vi "Notifier Release.vi"(8 "error in (no error)":errorcluster, 11 "Messaging in":refnum<class "Messaging.lvclass">) -> (0 "error out":errorcluster, 3 "Messaging out":refnum<class "Messaging.lvclass">)   [LabVIEW 2023, in "MessagingModule.lvlib" / "Messaging.lvclass"]
uses:
  Messaging.lvclass
  Messaging.lvclass/Messaging.ctl
  MessagingModule.lvlib
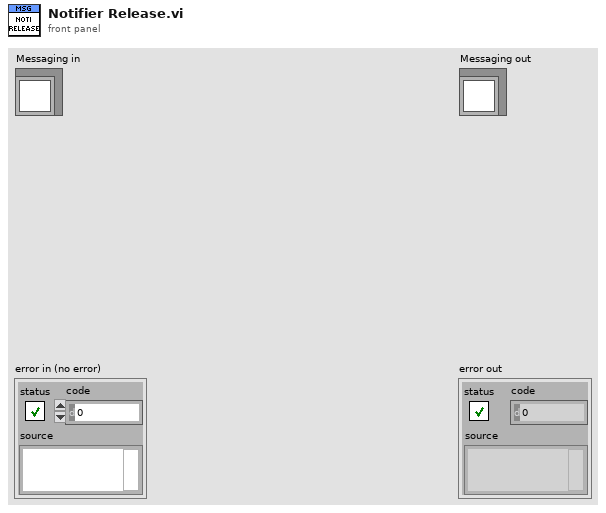
[diagram p1: front panel]
types:
  T1 = typedef "MessagingModule.lvlib/Msg.Noti.Ref.ctl" = refnum<notifier>
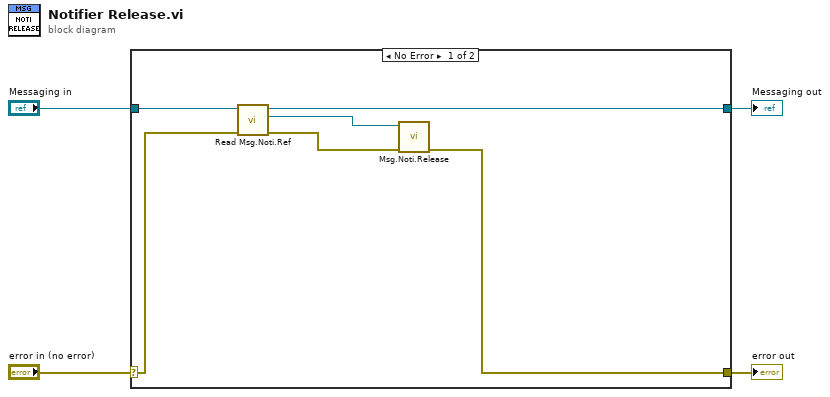
[diagram p0: block diagram]
diagram:
  n1 = case shown="No Error" "error in (no error)" {
    selector: "error in (no error)" -> [w9 w12]
    tunnel: [w6 w12] -> w3
    tunnel: [w8 w11] -> w1
    tunnel: "Messaging in" -> [w10 w11]
    frame No Error {
      n2 = call-dynamic "Read Msg.Noti.Ref.vi"("error in (no error)"=w9, "Messaging in"=w10) -> ("error out"=w7:errorcluster, "Msg.Noti.Ref"=w5:T1, "Messaging out"=w8:refnum<class "Messaging.lvclass">)  [unwired: 7 in]
      n3 = call "Msg.Noti.Release.vi"("Error (in)"=w7, "Msg.Noti.Ref"=w5) -> ("Error (out)"=w6:errorcluster)  [unwired: 9 in]
    }
    frame Error {
    }
  }
  "error out" <- w3
  "Messaging out" <- w1
